vi "H5Pisa_class.vi"(6 "error in (no error)":errorcluster, 8 "HDF5 Property List Class":T1, 9 "HDF5 Property List Ref":T1) -> (0 "error out":errorcluster, 2 "Member of class":bool, 3 "HDF5 Property List Ref out":T1)   [LabVIEW 2017]
doc: "Determines whether a property list is a member of a class."
uses:
  <vilib>/UPVI/lvhdf5/library.llb/HDF5 Ref.ctl
  <vilib>/UPVI/lvhdf5/hdf5.dll
panel:
  # "LVHDF5 Toolkit\nCopyright (c) 2005-2013 by Jason D. Sommerville\nCopyright (c) 2014 by UPVI, LLC.\n\nThis use and distribution of this file is governed by the terms found in \nLICENSE.txt distributed with this toolkit and installed at\n <user.lib>\\_lvhdf5\\LICENSE.txt"
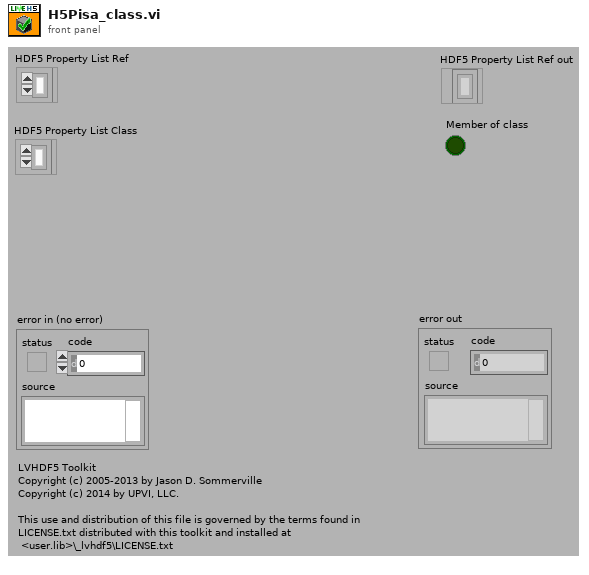
[diagram p1: front panel]
types:
  T1 = typedef "HDF5 Ref.ctl" = refnum<k1>
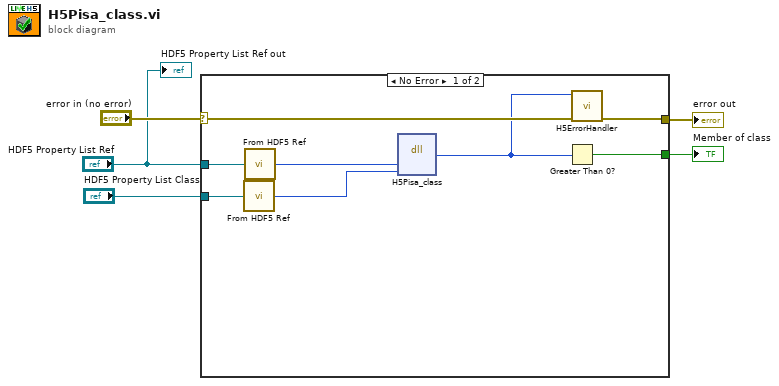
[diagram p0: block diagram]
diagram:
  n1 = case shown="No Error" "error in (no error)" {
    selector: "error in (no error)" -> [w13 w14]
    tunnel: [w12 w14] -> w4
    tunnel: "HDF5 Property List Ref" -> [w11 _]
    tunnel: "HDF5 Property List Class" -> [w9 _]
    tunnel: [w6 _] -> w1
    frame No Error {
      n2 = call <vilib>:"From HDF5 Ref.vi"("HDF5 Ref"=w9) -> ("I32"=w8:i32)
      n3 = call <vilib>:"From HDF5 Ref.vi"("HDF5 Ref"=w11) -> ("I32"=w10:i32)
      n4 = dll-call lib="C:/Program Files/National Instruments/LabVIEW 2017/vi.lib/UPVI/lvhdf5/hdf5.dll" fn="H5Pisa_class"("plist_id"=w10, "pclass"=w8) -> (w7:i32)  [unwired: 5 in, 2 out]
      n5 = Greater Than 0?(x=w7) -> (x > 0?=w6:bool)
      n6 = call <vilib>:"H5ErrorHandler.vi"("error in (no error)"=w13, "herr_t"=w7) -> ("error out"=w12:errorcluster)  [unwired: 3 in, 4 out]
    }
    frame Error {
    }
  }
  "error out" <- w4
  "Member of class" <- w1
  "HDF5 Property List Ref out" <- "HDF5 Property List Ref"
